vi "Insert Servicio in table.vi"(8 "error in (no error)":errorcluster, 10 "Servicio":string, 11 "Contabilidad in":refnum<class "Contabilidad.lvclass">) -> (0 "error out":errorcluster, 3 "Contabilidad out":refnum<class "Contabilidad.lvclass">)   [LabVIEW 2020, in "Contabilidad.lvlib" / "Contabilidad.lvclass"]
uses:
  Contabilidad.lvclass
  <vilib>/drjdpowell/SQLite Library/SQL Connection/Open (path).vi
  <vilib>/drjdpowell/SQLite Library/SQL Connection/Open (string).vi
  <vilib>/AdvancedString/Path To Command Line String.vi
  <vilib>/drjdpowell/SQLite Library/SQL Connection/Execute SQL (No results).vi
  <vilib>/drjdpowell/SQLite Library/SQL Connection/Connection.lvclass
  <vilib>/drjdpowell/SQLite Library/SQLite.lvlib
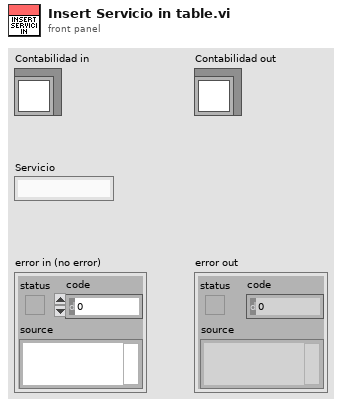
[diagram p1: front panel]
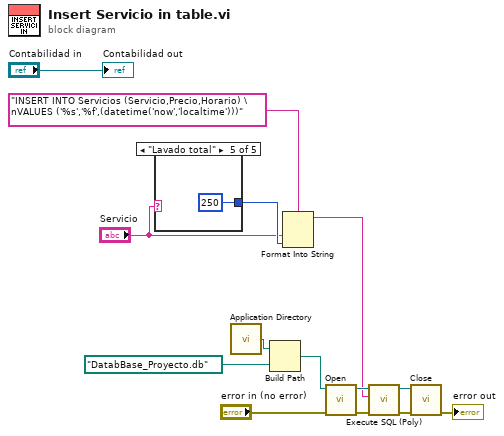
[diagram p0: block diagram]
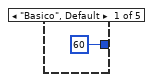
[diagram p2: hidden frame]
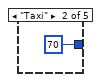
[diagram p3: hidden frame]
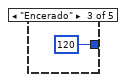
[diagram p4: hidden frame]
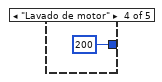
[diagram p5: hidden frame]
diagram:
  n1 = case shown="\"Lavado total\"" "Servicio" {
    tunnel: [60 70 120 200 250] -> w5
    frame "Basico", Default {
    }
    frame "Taxi" {
    }
    frame "Encerado" {
    }
    frame "Lavado de motor" {
    }
    frame "Lavado total" {
    }
  }
  n2 = call <vilib>:"Application Directory.vi"() -> ("Application Directory"=w10:path)
  n3 = Build Path(base path=w10, name or relative path=path "DatabBase_Proyecto.db") -> (appended path=w8:path)
  n4 = Format Into String(format string="INSERT INTO Servicios (Servicio,Precio,Horario) \nVALUES ('%s','%f',(datetime('now','localtime')))", "Servicio", w5) -> (resulting string=w1:string)  [unwired: 2 in, 1 out]
  n5 = call-poly <vilib>:"Open.vi"("error in (no error)"="error in (no error)", "db file"=w8) -> ("error out"=w12:errorcluster, "SQLite Connection"=w7:refnum<class "Connection.lvclass">)  [unwired: 8 in]
  n6 = call-poly <vilib>:"Execute SQL (Poly).vi"("error in (no error)"=w12, "SQL"=w1, "SQLite Connection in"=w7) -> ("error out"=w13:errorcluster, "SQLite Connection"=w6:refnum<class "Connection.lvclass">)  [unwired: 7 in]
  n7 = call-dynamic "Close.vi"("error in (no error)"=w13, "SQLite Connection in"=w6) -> ("error out"=→"error out":errorcluster)  [unwired: 9 in]
  "Contabilidad out" <- "Contabilidad in"
